vi "Filter_on_template_file_new.vi"(5 "Filetype":string, 6 "Filename":path, 7 "End Of File already Reached?":bool, 8 "Start of data (bytes)":i32, 9 "Data string":string, 10 "Channel Names In":string[](array[string]), 11 "Template File":path) -> (0 "Data Out":string[][](array[string]), 1 "Channel Names Out":string[](array[string]), 2 "Row numbers":i32[](array[numeric]), 3 "Template File-write":path, 4 "Deleted Rows":string[][](array[string]))   [LabVIEW 2015]
uses:
  Controls/Global_mode.ctl
panel:
  out "Current Case":string
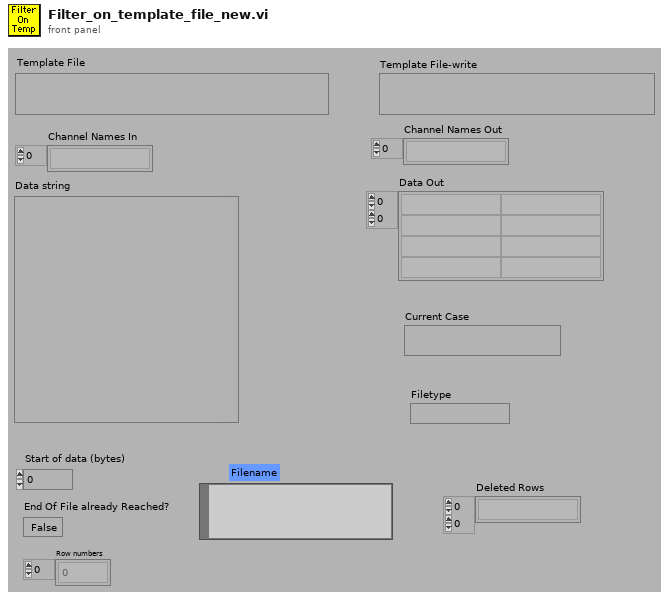
[diagram p1: front panel]
types:
  T1 = typedef "Global_mode.ctl" = enum16{"Read Global", "Load Global From File", "Write Global to File"}
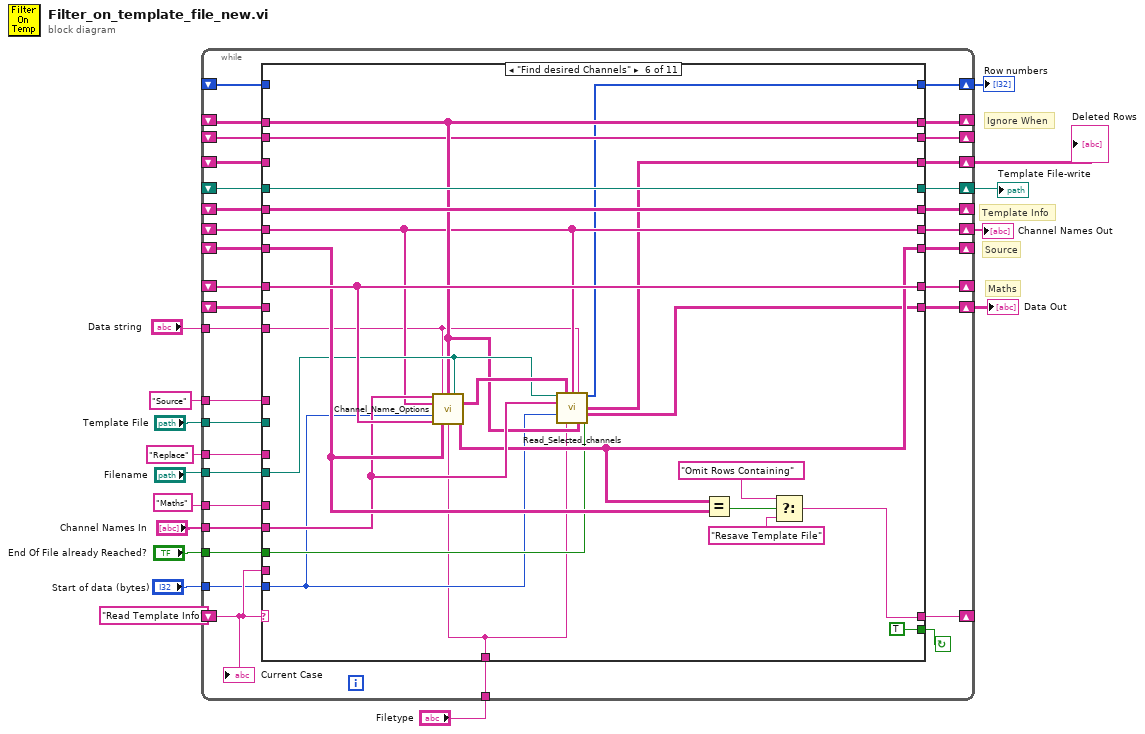
[diagram p0: block diagram]
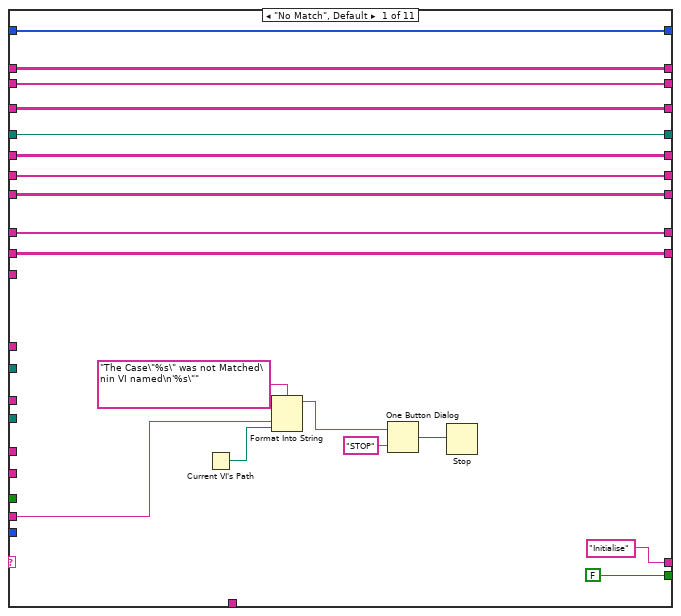
[diagram p2: hidden frame]
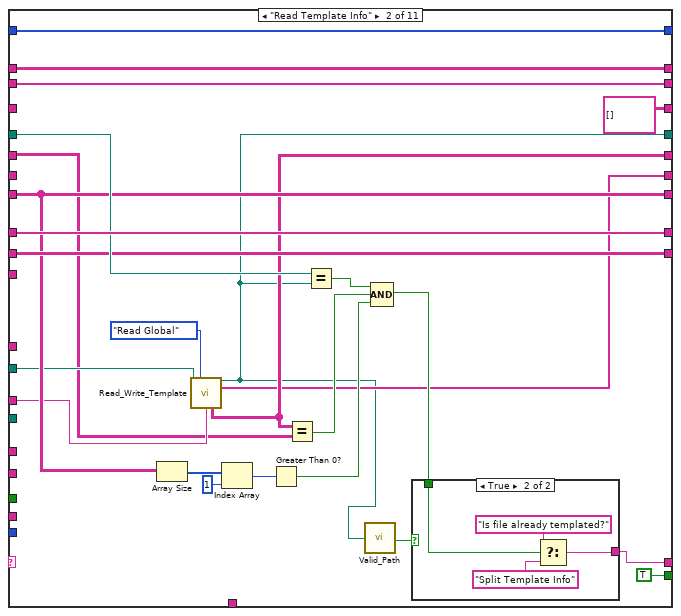
[diagram p3: hidden frame]
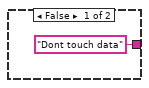
[diagram p4: hidden frame]
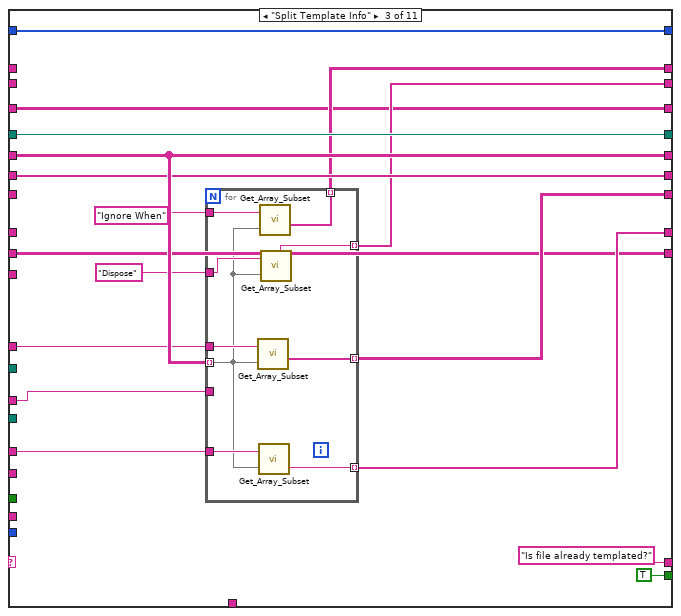
[diagram p5: hidden frame]
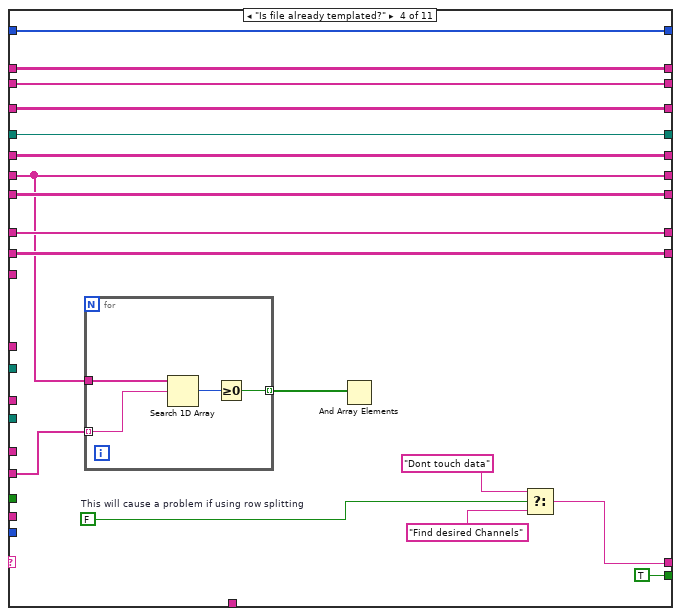
[diagram p6: hidden frame]
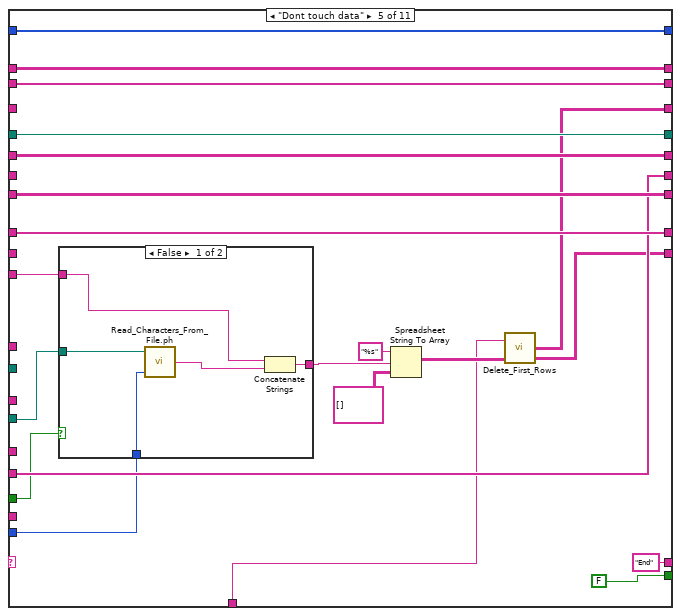
[diagram p7: hidden frame]
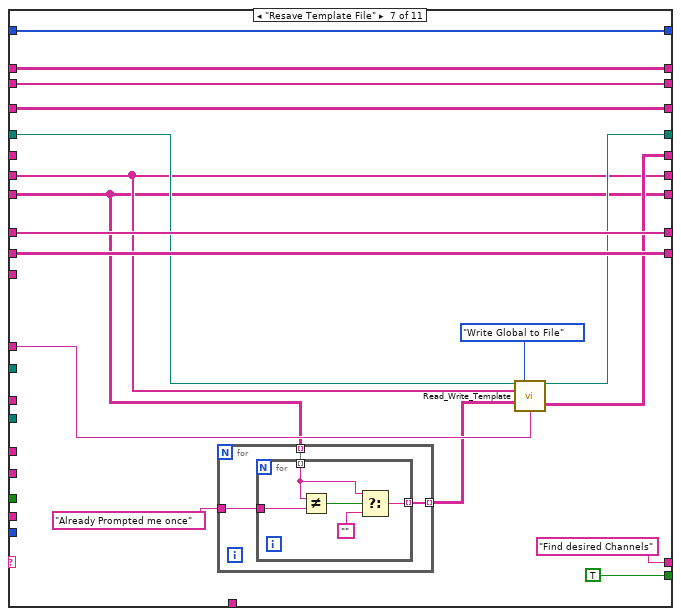
[diagram p9: hidden frame]
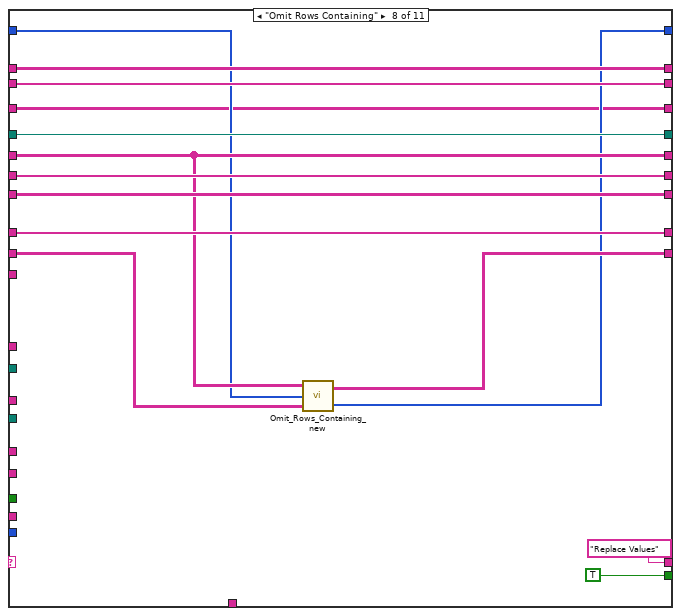
[diagram p10: hidden frame]
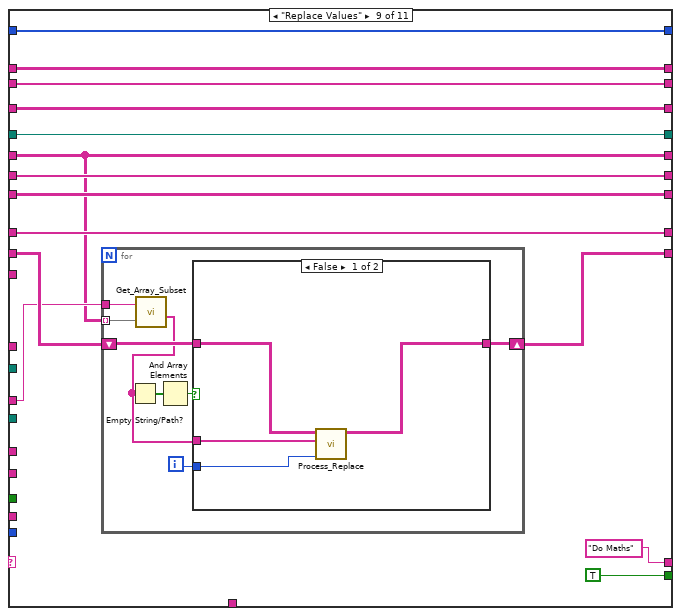
[diagram p11: hidden frame]
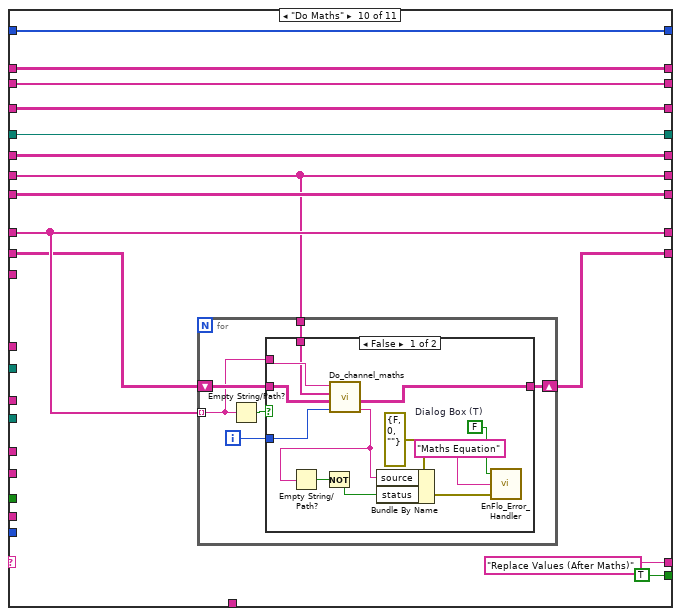
[diagram p13: hidden frame]
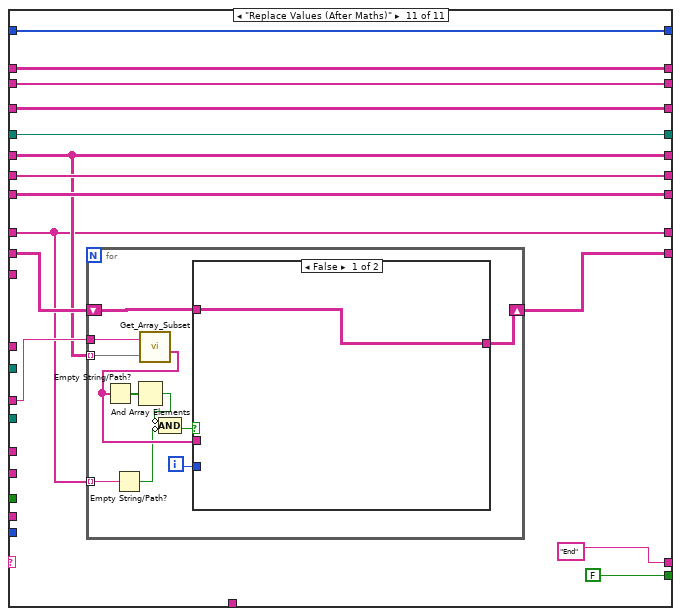
[diagram p15: hidden frame]
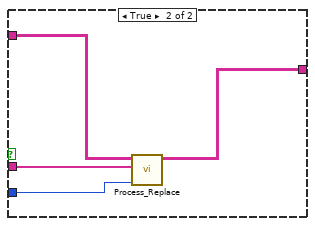
[diagram p16: hidden frame]
diagram:
  # "Ignore When"
  # "Maths"
  # "Template Info"
  # "Source"
  n1 = while {
    shift-left: _ -> [w21]
    shift-right: [w22] -> _
    tunnel: "Filetype" -> [w23]
    shift-left: _ -> [w25]
    shift-right: [w24] -> _
    tunnel: "Start of data (bytes)" -> [w26]
    tunnel: "Filename" -> [w28]
    tunnel: "End Of File already Reached?" -> [w29]
    tunnel: "Data string" -> [w30]
    tunnel: "Channel Names In" -> [w31]
    tunnel: "Template File" -> [w32]
    tunnel: "Maths" -> [w33]
    tunnel: "Replace" -> [w34]
    tunnel: "Source" -> [w35]
    shift-left: _ -> [w36]
    shift-right: [w37] -> w10
    shift-left: _ -> [w38]
    shift-right: [w39] -> _
    shift-left: _ -> [w40]
    shift-right: [w43] -> _
    shift-left: _ -> [w41]
    shift-right: [w44] -> w11
    shift-left: _ -> [w45]
    shift-right: [w46] -> _
    shift-left: _ -> [w42]
    shift-right: [w47] -> w15
    shift-left: "Read Template Info" -> [w27]
    shift-right: [w48] -> _
    shift-right: [w19] -> w2
    shift-left: _ -> [w20]
    shift-right: [w18] -> w1
    shift-left: _ -> [w17]
    stop <- w49 continue-if-true
    n2 = case shown="\"Find desired Channels\"" w27 {
      tunnel: [FALSE TRUE TRUE TRUE ("Duplicate rows?") FALSE ("Duplicate rows?") TRUE TRUE TRUE TRUE TRUE ("Duplicate rows?") FALSE] -> w49
      tunnel: ["Initialise" w90 "Is file already templated?" w132 "End" w193 "Find desired Channels" "Replace Values" "Do Maths" "Replace Values (After Maths)" "End"] -> w48
      tunnel: w27 -> [w62 _ _ _ _ _ _ _ _ _ _]
      tunnel: [w59 w70 w112 w140 w165 w192 w205 w228 w243 w272 w303] -> w47
      tunnel: [w58 w77 w113 w136 w162 w191 w203 w227 w235 w271 w295] -> w46
      tunnel: w45 -> [w58 w76 w113 w136 w162 w191 _ w227 w235 w271 w295]
      tunnel: [w57 w72 w106 w128 w159 w181 w202 w231 w240 w265 w300] -> w44
      tunnel: [w56 w81 w110 w139 w164 w187 w198 w229 w244 w273 w304] -> w43
      tunnel: w42 -> [w59 w86 w112 w140 w165 w192 w204 w228 w243 w272 w303]
      tunnel: w41 -> [w57 _ w106 w128 _ w181 w202 w231 w240 w265 w300]
      tunnel: w40 -> [w56 w81 _ w139 w164 w189 w198 w229 w244 w273 w304]
      tunnel: [w55 w87 w111 w138 w163 w190 w209 w230 w245 w270 w294] -> w39
      tunnel: w38 -> [w55 w87 _ w138 w163 w190 w209 w230 w245 w270 w294]
      tunnel: [w54 w85 w109 w137 w149 w182 w208 w225 w242 w266 w302] -> w37
      tunnel: w36 -> [w54 w85 w109 w137 _ _ w208 w226 w241 w267 w301]
      tunnel: w35 -> [_ _ w108 _ _ _ w206 _ _ _ _]
      tunnel: w34 -> [_ w78 w104 _ _ _ _ _ w236 _ w296]
      tunnel: w33 -> [_ _ w107 _ _ _ _ _ _ _ _]
      tunnel: w32 -> [_ w79 _ _ _ _ _ _ _ _ _]
      tunnel: w31 -> [_ _ _ w130 w159 w188 _ _ _ _ _]
      tunnel: w30 -> [_ _ _ _ w153 w177 _ _ _ _ _]
      tunnel: w29 -> [_ _ _ _ w156 w185 _ _ _ _ _]
      tunnel: w28 -> [_ _ _ _ w155 w184 _ _ _ _ _]
      tunnel: w26 -> [_ _ _ _ w154 w179 _ _ _ _ _]
      tunnel: [w53 w74 w103 w129 w151 w180 w201 w224 w239 w264 w299] -> w24
      tunnel: w25 -> [w53 w74 _ w129 w151 w180 w201 w224 w239 w264 w299]
      tunnel: w23 -> [_ _ _ _ w148 w178 _ _ _ _ _]
      tunnel: [w52 w73 w100 w127 w147 w183 w200 w223 w238 w263 w298] -> w22
      tunnel: w21 -> [w52 w73 _ w127 w147 w183 w200 w223 w238 w263 w298]
      tunnel: [w51 w71 w99 w125 w146 w174 w196 w222 w237 w262 w297] -> w19
      tunnel: w20 -> [w51 w71 w99 w125 w146 _ w196 w221 w237 w262 w297]
      tunnel: [w50 string[][] [] ("Deleted Rows") w98 w124 w145 w172 w195 w220 w234 w261 w293] -> w18
      tunnel: w17 -> [w50 _ w98 w124 _ _ w195 w220 w234 w261 w293]
      frame "No Match", Default {
        n3 = Current VI's Path() -> (path=w61:path)
        n4 = Format Into String(format string="The Case\"%s\" was not Matched\nin VI named\n'%s\"" ("Format String"), w62, w61) -> (resulting string=w65:string)  [unwired: 2 in, 1 out]
        n5 = One Button Dialog(message=w65, button name ("OK")="STOP") -> (true=w63:bool)
        n6 = Stop(stop? (T)=w63) -> ()
      }
      frame "Read Template Info" {
        n7 = Array Size(array=w81) -> (size(s)=w84:i32[])
        n8 = call "Read_Write_Template.vi"("Template File"=w79, "Mode"=Global_mode."Read Global", "Data type"=w78) -> ("Template File Out"=w70:path, "Template Ch Names Out"=w72:string[], "Template Info"=w77:string[][])  [unwired: 5 in, 5 out]
        n9 = Index Array(array=w84, index=1 ("Index")) -> (element=w82:i32)
        n10 = Greater Than 0?(x=w82) -> (x > 0?=w80:bool)
        n11 = Equal?(x=w77, y=w76) -> (x = y?=w75:bool)
        n12 = Equal?(x=w86, y=w70) -> (x = y?=w89:bool)
        n13 = call "Valid_Path.vi"("Filename"=w70) -> ("Valid Path?"=w69:bool)
        n14 = Compound Arithmetic op=AND(w89, w75, w80) -> (w88:bool)
        n15 = case shown="True" w69 {
          tunnel: ["Dont touch data" w97] -> w90
          tunnel: w88 -> [_ w94]
          frame False {
          }
          frame True {
            n16 = Select(t="Is file already templated?", s=w94, f="Split Template Info") -> (s? t:f=w97:string)
          }
        }
      }
      frame "Split Template Info" {
        n17 = for {
          tunnel: w113 -> [w116] mode=indexing
          tunnel: w108 -> [w123]
          tunnel: w107 -> [w122]
          tunnel: [w121] -> w110 mode=indexing
          tunnel: [w120] -> w111 mode=indexing
          tunnel: w104 -> [_]
          tunnel: [w119] -> w103 mode=indexing
          tunnel: "Dispose" -> [w118]
          tunnel: "Ignore When" -> [w117]
          tunnel: [w115] -> w100 mode=indexing
          n18 = call "Get_Array_Subset.vi"("String Array In"=w116, "Subset Name"=w123) -> ("Array Subset Out"=w121:string[])  [unwired: 4 out]
          n19 = call "Get_Array_Subset.vi"("String Array In"=w116, "Subset Name"=w122) -> ("First Element"=w120:string)  [unwired: 4 out]
          n20 = call "Get_Array_Subset.vi"("String Array In"=w116, "Subset Name"=w117) -> ("Array Subset Out"=w115:string[])  [unwired: 4 out]
          n21 = call "Get_Array_Subset.vi"("String Array In"=w116, "Subset Name"=w118) -> ("First Element"=w119:string)  [unwired: 4 out]
        }
      }
      frame "Is file already templated?" {
        w126 = FALSE  # This will cause a problem if using row splitting
        n22 = for {
          tunnel: [w144] -> w131 mode=indexing
          tunnel: w128 -> [w142]
          tunnel: w130 -> [w141] mode=indexing
          n23 = Search 1D Array(1D array=w142, element=w141) -> (index of element=w143:i32)  [unwired: 1 out]
          n24 = Greater Or Equal To 0?(x=w143) -> (x >= 0?=w144:bool)
        }
        n25 = And Array Elements(Boolean array=w131) -> ()  [unwired: 1 out]
        n26 = Select(t="Dont touch data", s=w126, f="Find desired Channels") -> (s? t:f=w132:string)
      }
      frame "Dont touch data" {
        n27 = case shown="False" w156 {
          tunnel: w155 -> [w169 _]
          tunnel: w154 -> [w168 _]
          tunnel: w153 -> [w167 w171]
          tunnel: [w166 w171] -> w152
          frame False {
            n28 = call "Read_Characters_From_File.ph.vi"("file path (dialog if empty)"=w169, "start of read offset (chars.: 0)"=w168) -> ("character string"=w170:string)  [unwired: 1 in, 6 out]
            n29 = Concatenate Strings(w167, w170) -> (w166:string)
          }
          frame True {
          }
        }
        n30 = Spreadsheet String To Array(format string="%s", spreadsheet string=w152, array type (2D Dbl)=string[][] [] ("Channel Values")) -> (array=w150:string[][])  [unwired: 1 out]
        n31 = call "Delete_First_Rows.vi"("File Type"=w148, "Data In"=w150) -> ("Deleted Rows"=w145:string[][], "Data Out"=w149:string[][])  [unwired: 1 out]
      }
      frame "Find desired Channels" {
        n32 = call "Channel_Name_Options.vi"("All Channel Names"=w188, "Data string"=w177, "Ignore When"=w183, "Reading Filename"=w184, "Template Names"=w181, "Start of data (bytes)"=w179, "Maths In"=w190, "Name Options In"=w189, "Filetype"=w178) -> ("Valid Channel Options"=w186:string[][], "Name Options Out"=w187:string[][])  [unwired: 2 in, 3 out]
        n33 = call "Read_Selected_channels.vi"("Filename"=w184, "Valid Channel Options"=w186, "Template Names"=w181, "Data string"=w177, "All Channels Present"=w188, "End Of File already Reached?"=w185, "Start of data (bytes)"=w179, "Filetype"=w178, "Ignore When"=w183) -> ("Non-Blank Rows"=w174:i32[], "Deleted Rows"=w172:string[][], "Output Values"=w182:string[][])  [unwired: 2 in, 2 out]
        n34 = Equal?(x=w187, y=w189) -> (x = y?=w175:bool)
        n35 = Select(t="Omit Rows Containing", s=w175, f="Resave Template File") -> (s? t:f=w193:string)
      }
      frame "Resave Template File" {
        n36 = for {
          tunnel: "Already Prompted me once" -> [w214]
          tunnel: w198 -> [w213] mode=indexing
          tunnel: [w212] -> w197 mode=indexing
          n37 = for {
            tunnel: w214 -> [w219]
            tunnel: w213 -> [w217] mode=indexing
            tunnel: [w215] -> w212 mode=indexing
            n38 = Not Equal?(x=w217, y=w219) -> (x != y?=w218:bool)
            n39 = Select(t=w217, s=w218, f="") -> (s? t:f=w215:string)
          }
        }
        n40 = call "Read_Write_Template.vi"("Template File"=w204, "Mode"=Global_mode."Write Global to File", "Channel names In"=w202, "2D Info In"=w197, "Data type"=w206) -> ("Template File Out"=w205:path, "Template Info"=w203:string[][])  [unwired: 3 in, 6 out]
      }
      frame "Omit Rows Containing" {
        n41 = call "Omit_Rows_Containing_new.vi"("Data Array In"=w226, "Non-Blank Rows"=w221, "Template Info"=w227) -> ("Row numbers"=w222:i32[], "Data Array Out"=w225:string[][])
      }
      frame "Replace Values" {
        n42 = for {
          shift-right: [w253] -> w242
          shift-left: w241 -> [w254]
          tunnel: w236 -> [w250]
          tunnel: w235 -> [w249] mode=indexing
          i -> [w255]
          n43 = call "Get_Array_Subset.vi"("String Array In"=w249, "Subset Name"=w250) -> ("Array Subset Out"=w248:string[])  [unwired: 4 out]
          n44 = Empty String/Path?(string/path=w248) -> (empty?=w252:bool[])
          n45 = And Array Elements(Boolean array=w252) -> (logical AND=w251:bool)
          n46 = case shown="False" w251 {
            tunnel: w248 -> [w259 _]
            tunnel: w255 -> [w256 _]
            tunnel: w254 -> [w258 w260]
            tunnel: [w257 w260] -> w253
            frame False {
              n47 = call "Process_Replace.vi"("Index"=w256, "Replace array"=w259, "Array In"=w258) -> ("Array Out"=w257:string[][])  [unwired: 1 in, 3 out]
            }
            frame True {
            }
          }
        }
      }
      frame "Do Maths" {
        n48 = for {
          tunnel: w270 -> [w275] mode=indexing
          shift-right: [w277] -> w266
          shift-left: w267 -> [w276]
          tunnel: w265 -> [w274]
          i -> [w278]
          n49 = Empty String/Path?(string/path=w275) -> (empty?=w279:bool)
          n50 = case shown="False" w279 {
            tunnel: w278 -> [w291 _]
            tunnel: [w289 w292] -> w277
            tunnel: w276 -> [w290 w292]
            tunnel: w275 -> [w288 _]
            tunnel: w274 -> [w287 _]
            frame False {
              w280 = FALSE  # Dialog Box (T)
              n51 = call "Do_channel_maths.vi"("Output Index"=w291, "Channel Values In"=w290, "Channel Names"=w287, "Maths Equation"=w288) -> ("Error String"=w284:string, "Channel Values Out"=w289:string[][])  [unwired: 2 out]
              n52 = Empty String/Path?(string/path=w284) -> (empty?=w286:bool)
              n53 = Not(x=w286) -> (.not. x?=w283:bool)
              n54 = Bundle By Name(cluster=errorcluster {"status"=FALSE, "code"=0, "source"=""} ("error in (no error)"), "source"=w284, "status"=w283) -> (w282:errorcluster)
              n55 = call "EnFlo_Error_Handler.vi"("error in (no error)"=w282, "Error Type"="Maths Equation", "Dialog Box (T)"=w280) -> ()  [unwired: 3 out]
            }
            frame True {
            }
          }
        }
      }
      frame "Replace Values (After Maths)" {
        n56 = for {
          shift-right: [w315] -> w302
          shift-left: w301 -> [w316]
          tunnel: w296 -> [w313]
          tunnel: w295 -> [w312] mode=indexing
          tunnel: w294 -> [w308] mode=indexing
          i -> [w317]
          n57 = Empty String/Path?(string/path=w308) -> (empty?=w307:bool)
          n58 = call "Get_Array_Subset.vi"("String Array In"=w312, "Subset Name"=w313) -> ("Array Subset Out"=w311:string[])  [unwired: 4 out]
          n59 = Empty String/Path?(string/path=w311) -> (empty?=w314:bool[])
          n60 = And Array Elements(Boolean array=w314) -> (logical AND=w310:bool)
          n61 = Compound Arithmetic op=AND(invert w310, invert w307) -> (w309:bool)
          n62 = case shown="False" w309 {
            tunnel: w311 -> [_ w322]
            tunnel: w317 -> [_ w319]
            tunnel: w316 -> [w318 w321]
            tunnel: [w318 w320] -> w315
            frame False {
            }
            frame True {
              n63 = call "Process_Replace.vi"("Index"=w319, "Replace array"=w322, "Array In"=w321) -> ("Array Out"=w320:string[][])  [unwired: 1 in, 3 out]
            }
          }
        }
      }
    }
    "Current Case" <- w27
  }
  "Channel Names Out" <- w11
  "Data Out" <- w10
  "Template File-write" <- w15
  "Row numbers" <- w2
  "Deleted Rows" <- w1
